vi "TCP-error-int.vi"(8 "error in (no error)":errorcluster, 10 "Retun code":u32) -> (0 "error out":errorcluster)   [LabVIEW 2013, in "EC1000-control.lvlib" / "SM1000-control.lvclass"]
doc: "Verified if the return string contains at least the \nexpected string. Case insensitive."
uses:
  SM1000-control.lvclass
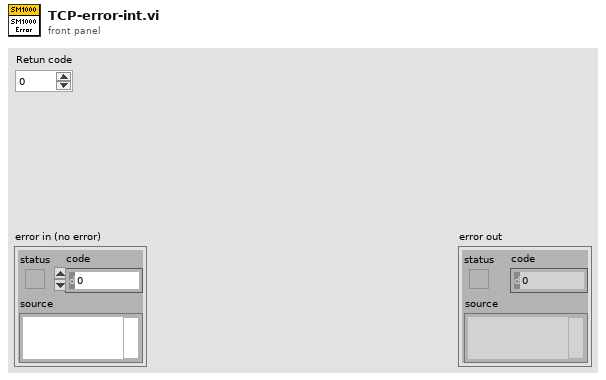
[diagram p1: front panel]
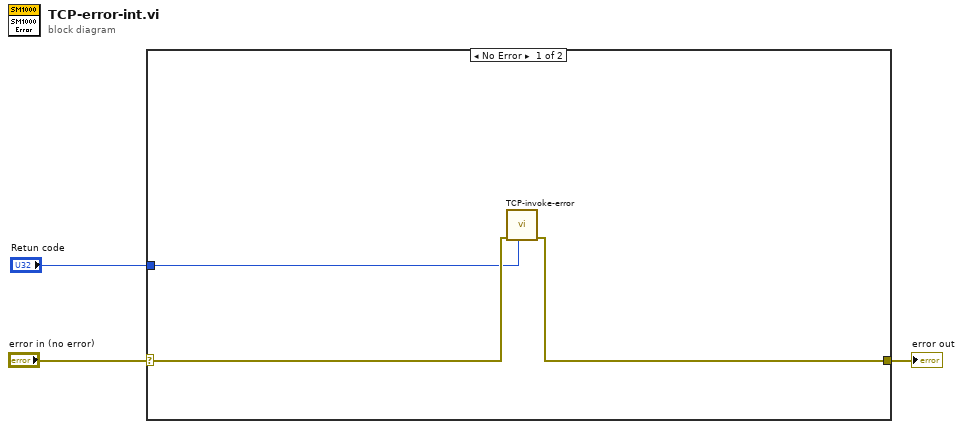
[diagram p0: block diagram]
diagram:
  n1 = case shown="No Error" "error in (no error)" {
    selector: "error in (no error)" -> [w6 w7]
    tunnel: [w4 w7] -> w2
    tunnel: "Retun code" -> [w5 _]
    frame No Error {
      n2 = call "TCP-invoke-error.vi"("Return-code"=w5, "error in (no error)"=w6) -> ("error out"=w4:errorcluster)  [unwired: 9 in]
    }
    frame Error {
    }
  }
  "error out" <- w2
